vi "FPGAoutput_from_DDS_to_host.vi"() -> ()   [LabVIEW 2013]
uses:
  Input_5782/5782_states.ctl
  <vilib>/Platform/TimedLoop/XDataNode/timing_clust.ctl
  <vilib>/Platform/TimedLoop/XDataNode/nitl_modes.ctl
  <vilib>/Platform/TimedLoop/XDataNode/wakeup.ctl
  <vilib>/rvi/Emulation/niFpgaSctlEmulationGetInTimedLoop.vi
  <vilib>/rvi/Emulation/niFpgaEmulationReportErrorSimple.vi
  <vilib>/rvi/Emulation/niFpgaGetClockAttributes.vi
  <vilib>/rvi/Emulation/niFpgaCriticalErrorInLSC.vi
  <vilib>/rvi/interface/RandomDataEmulation/nirviRandomDataMultiElementFPGAFIFO.vi
  <instcachedir>/0/nirviRandomDataMultiElementFPGAFIFO_F2B80EDE0D7944A08478D8D26097D4DB.lvgen/nirviRandomDataMultiElementFPGAFIFO_F2B80EDE0D7944A08478D8D26097D4DB_005.vi
  <vilib>/rvi/interface/RandomDataEmulation/niFpgaRandomDataHandleErrors.vi
  <vilib>/Platform/TimedLoop/XDataNode/XDataNode.xnode
  <vilib>/rvi/FXPMathLib/FxpInterpret/XNode/nifxpmath_Interpret.xnode
  <vilib>/rvi/DataTransferAndStorage/Container/XNode/niFpgaContainer.xnode
  <vilib>/rvi/interface/RandomDataEmulation/nirviRandomDataFpgaMultiElementTemplate.vi
  <vilib>/Platform/TimedLoop/XDataNode/XDNodeRunTimeDep.lvlib
panel:
  in  "5782 record length":u16=4000 caption="Samples Per Trigger" min=1 step=1
  in  "Trigger Acquisition":bool
  in  "Phase output":fxp<+,64,64>[](array[numeric])=[0.0, 0.0, 0.0, 0.0, 0.0, 0.0, 0.0, 0.0]
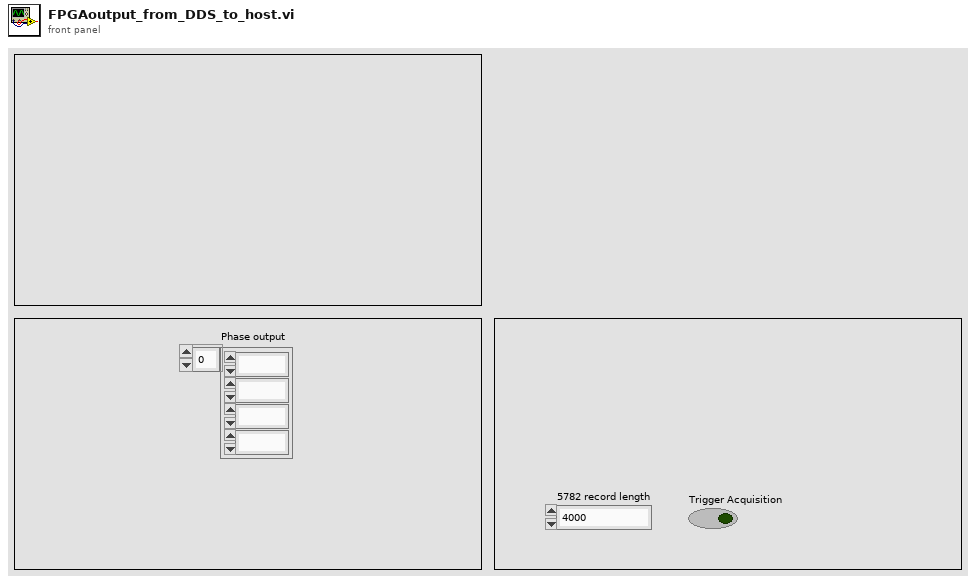
[diagram p1: front panel]
types:
  T1 = typedef "5782_states.ctl" = enum8{"Wait for trigger", "Acquisition", "Send record length", "Quiet period"}
  T2 = typedef "XDNodeRunTimeDep.lvlib/timing_clust.ctl" = cluster{"Expected End [f-1]":u64, "Actual End [f-1]":u64, "Finished Late? [f-1]":bool, "Expected End [i-1]":u64, "Actual End [i-1]":u64, "Finished Late? [i-1]":bool, "Expected Start [i]":u64, "Actual Start [i]":u64, "Expected Start [f]":u64, "Actual Start [f]":u64, "Source Name":string, "Structure Name":string, "Period":i64, "Deadline":i64, "Offset":i64, "Start":i64, "Priority":i32, "Timeout":i32, "Mode":T3, "Wakeup Reason":T4, "Error":errorcluster, "Source Type":string, "Secondary Source Type":string, "Global End Time":u64, "Global Start Time":u64, "Frame Duration":u64, "Iteration Duration":u64, "Assigned CPU":i32, "I/O Scan Engine Mode":u32}
  T3 = typedef "XDNodeRunTimeDep.lvlib/nitl_modes.ctl" = enum32{"No Change", "Process missed periods, maintain original phase", "Discard missed periods, maintain original phase", "Process missed periods, ignore original phase", "Discard missed periods, ignore original phase"}
  T4 = typedef "XDNodeRunTimeDep.lvlib/wakeup.ctl" = enum32{"Normal", "Aborted", "Asynchronous wakeup", "Timing source error", "Timed loop error", "Timeout"}
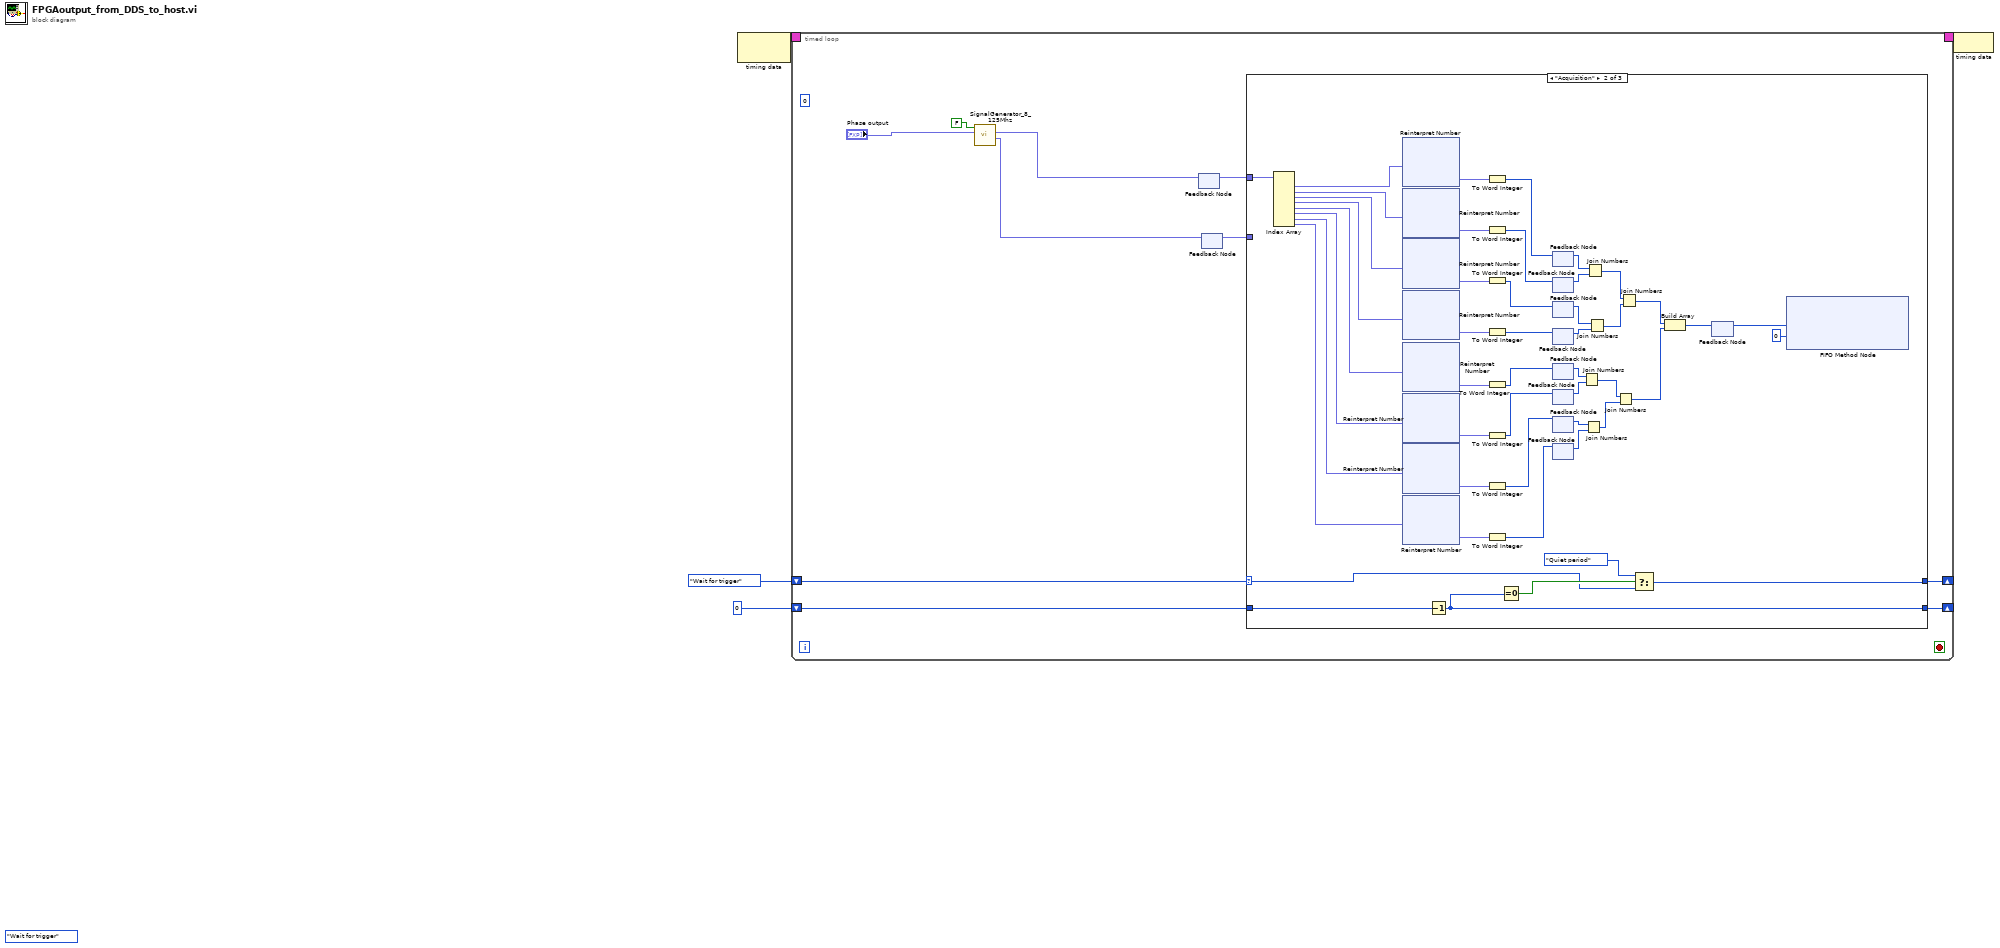
[diagram p0: block diagram]
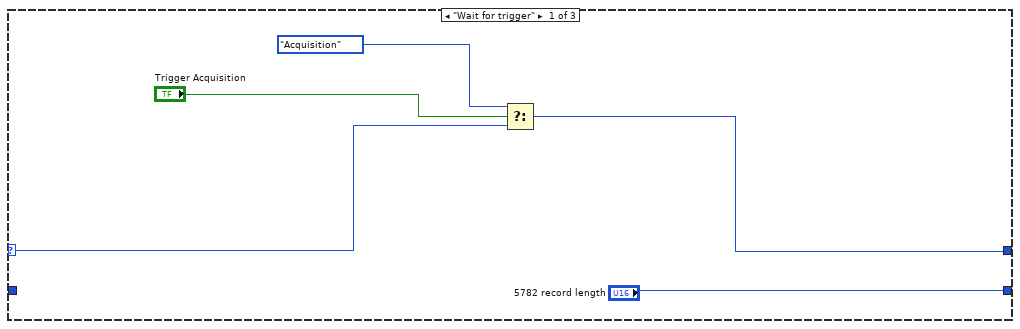
[diagram p2: hidden frame]
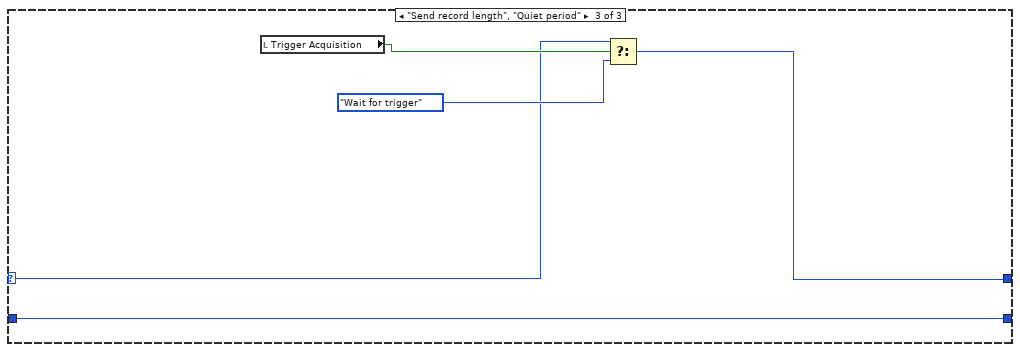
[diagram p3: hidden frame]
diagram:
  (unwired) 5782_states."Wait for trigger" ("5782 states")
  n1 = node-c288() -> (w4:T2)  [unwired: 1 in]
  n2 = timed-loop {
    timing: w4 -> [_]
    timing-out: [_] -> w3
    shift-right: [w9] -> _
    shift-left: 5782_states."Wait for trigger" ("5782 states") -> [w10]
    shift-right: [w8] -> _
    shift-left: u16 0 ("5782 record length") -> [w7]
    stop <- _ stop-if-true
    (unwired) 0 ("Timeout")
    n3 = call "SignalGenerator_8_125Mhz.vi"("Phase"="Phase output", "reset"=FALSE) -> ("Sine out"=w6:fxp<+/-,16,0>[], "Cosine out"=w11:fxp<+/-,16,0>[])  [unwired: 8 in]
    n4 = feedback #1() -> (w12:fxp<+/-,16,0>[])  [unwired: 1 in]
    n5 = feedback-in #1(w11) -> ()
    n6 = feedback #2() -> (w5:fxp<+/-,16,0>[])  [unwired: 1 in]
    n7 = feedback-in #2(w6) -> ()
    n8 = case shown="\"Acquisition\"" w10 {
      selector: w10 -> [w18 w20 w70]
      tunnel: w12 -> [_ w67 _]
      tunnel: [w17 w24 w69] -> w9
      tunnel: ["5782 record length" w25 w68] -> w8
      tunnel: w7 -> [_ w27 w68]
      tunnel: w5 -> [_ _ _]
      frame "Wait for trigger" {
        n9 = Select(t=5782_states."Acquisition" ("5782 states"), s="Trigger Acquisition", f=w18) -> (s? t:f=w17:T1)
      }
      frame "Acquisition" {
        n10 = Index Array(array=w67) -> (element #1=w64:fxp<+/-,16,0>, element #2=w49:fxp<+/-,16,0>, element #3=w48:fxp<+/-,16,0>, element #4=w47:fxp<+/-,16,0>, element #5=w46:fxp<+/-,16,0>, element #6=w45:fxp<+/-,16,0>, element #7=w44:fxp<+/-,16,0>, element #8=w43:fxp<+/-,16,0>)  [unwired: 8 in]
        n11 = xnode "Reinterpret Number"("x"=w64) -> ("y"=w66:fxp<+/-,16,16>)
        n12 = xnode "Reinterpret Number"("x"=w49) -> ("y"=w63:fxp<+/-,16,16>)
        n13 = xnode "Reinterpret Number"("x"=w48) -> ("y"=w62:fxp<+/-,16,16>)
        n14 = xnode "Reinterpret Number"("x"=w47) -> ("y"=w61:fxp<+/-,16,16>)
        n15 = xnode "Reinterpret Number"("x"=w46) -> ("y"=w57:fxp<+/-,16,16>)
        n16 = xnode "Reinterpret Number"("x"=w45) -> ("y"=w58:fxp<+/-,16,16>)
        n17 = xnode "Reinterpret Number"("x"=w44) -> ("y"=w59:fxp<+/-,16,16>)
        n18 = xnode "Reinterpret Number"("x"=w43) -> ("y"=w60:fxp<+/-,16,16>)
        n19 = Decrement(x=w27) -> (x-1=w25:u16)
        n20 = To Word Integer(number=w66) -> (16bit integer=w65:i16)
        n21 = To Word Integer(number=w63) -> (16bit integer=w56:i16)
        n22 = To Word Integer(number=w62) -> (16bit integer=w55:i16)
        n23 = To Word Integer(number=w61) -> (16bit integer=w54:i16)
        n24 = To Word Integer(number=w57) -> (16bit integer=w53:i16)
        n25 = To Word Integer(number=w58) -> (16bit integer=w52:i16)
        n26 = To Word Integer(number=w59) -> (16bit integer=w51:i16)
        n27 = To Word Integer(number=w60) -> (16bit integer=w50:i16)
        n28 = Equal To 0?(x=w25) -> (x = 0?=w26:bool)
        n29 = feedback #3() -> (w42:i16)  [unwired: 1 in]
        n30 = feedback-in #3(w65) -> ()
        n31 = feedback #4() -> (w41:i16)  [unwired: 1 in]
        n32 = feedback-in #4(w56) -> ()
        n33 = feedback #5() -> (w40:i16)  [unwired: 1 in]
        n34 = feedback-in #5(w55) -> ()
        n35 = feedback #6() -> (w39:i16)  [unwired: 1 in]
        n36 = feedback-in #6(w54) -> ()
        n37 = feedback #7() -> (w38:i16)  [unwired: 1 in]
        n38 = feedback-in #7(w53) -> ()
        n39 = feedback #8() -> (w36:i16)  [unwired: 1 in]
        n40 = feedback-in #8(w52) -> ()
        n41 = feedback #9() -> (w37:i16)  [unwired: 1 in]
        n42 = feedback-in #9(w51) -> ()
        n43 = feedback #10() -> (w35:i16)  [unwired: 1 in]
        n44 = feedback-in #10(w50) -> ()
        n45 = Join Numbers(hi=w38, lo=w36) -> ((hi.lo)=w32:u32)
        n46 = Join Numbers(hi=w37, lo=w35) -> ((hi.lo)=w31:u32)
        n47 = Join Numbers(hi=w42, lo=w41) -> ((hi.lo)=w34:u32)
        n48 = Join Numbers(hi=w40, lo=w39) -> ((hi.lo)=w33:u32)
        n49 = Join Numbers(hi=w32, lo=w31) -> ((hi.lo)=w29:u64)
        n50 = Join Numbers(hi=w34, lo=w33) -> ((hi.lo)=w30:u64)
        n51 = Select(t=5782_states."Quiet period" ("5782 states"), s=w26, f=w20) -> (s? t:f=w24:T1)
        n52 = Build Array(w30, w29) -> (w23:u64[])
        n53 = feedback #11() -> (w22:u64[])  [unwired: 1 in]
        n54 = feedback-in #11(w23) -> ()
        n55 = xnode ("FIFO Method Node")("Element"=w22, "Timeout"=0) -> ()  [unwired: 1 in, 2 out]
      }
      frame "Send record length", "Quiet period" {
        n56 = local read "Trigger Acquisition"() -> (w72:bool)
        n57 = Select(t=w70, s=w72, f=5782_states."Wait for trigger" ("5782 states")) -> (s? t:f=w69:T1)
      }
    }
  }
  n58 = node-c288(w3) -> ()
